vi "REAL worker.vi"(3 "channel":i8) -> (1 "Action running":T1(ring)=enum."pre-reaction")   [LabVIEW 2023]
panel:
  out "Time/min":i32
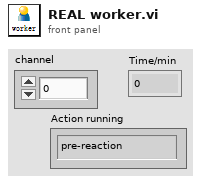
[diagram p1: front panel]
types:
  T1 = enum16{"standby", "pre-reaction", "reaction", "post-reaction", "analysis"}
  T2 = enum16{"check", "scan", "index", "read", "add", "write"}
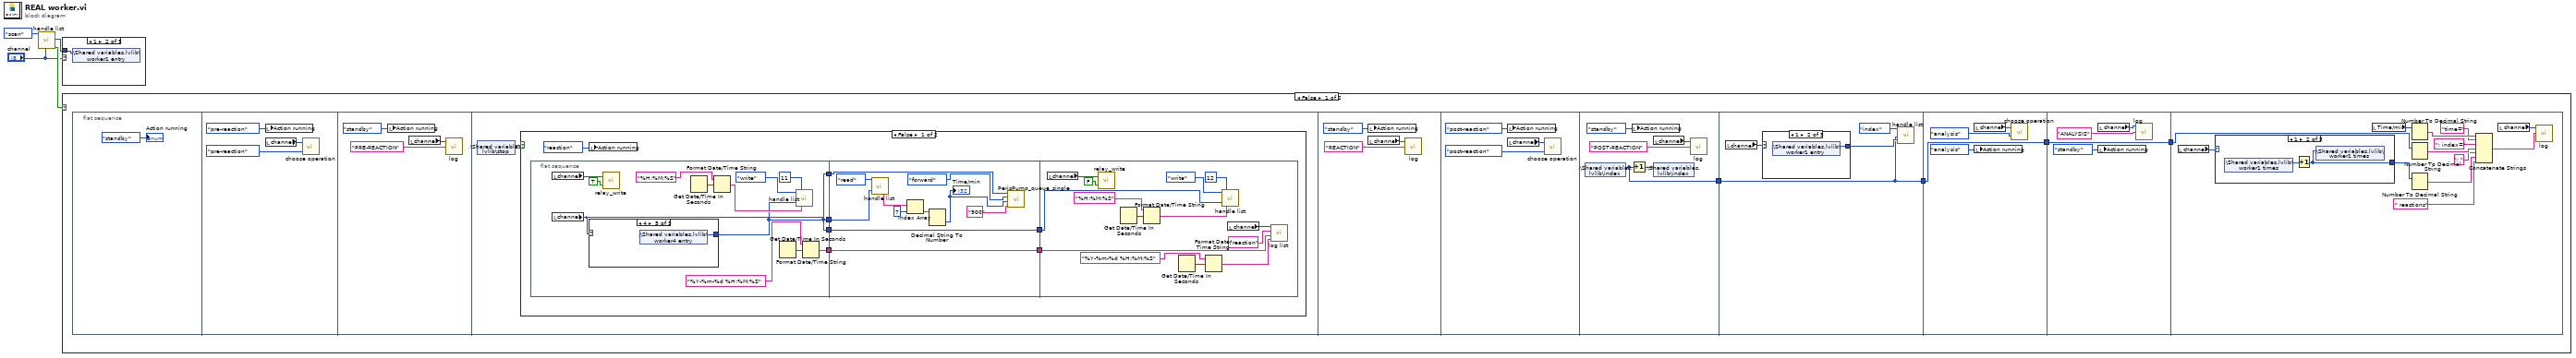
[diagram p0: block diagram]
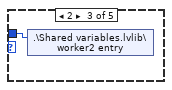
[diagram p3: hidden frame]
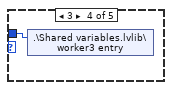
[diagram p4: hidden frame]
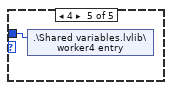
[diagram p5: hidden frame]
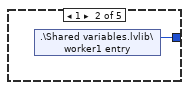
[diagram p7: hidden frame]
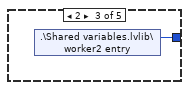
[diagram p8: hidden frame]
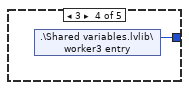
[diagram p9: hidden frame]
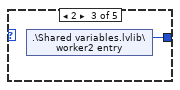
[diagram p12: hidden frame]
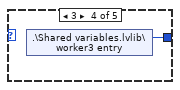
[diagram p13: hidden frame]
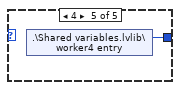
[diagram p14: hidden frame]
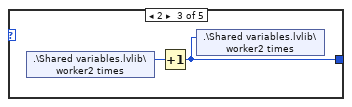
[diagram p16: hidden frame]
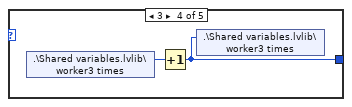
[diagram p17: hidden frame]
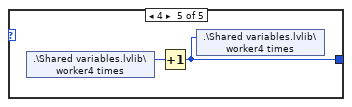
[diagram p18: hidden frame]
diagram:
  n1 = call "handle list.vi"("operation"=T2."scan", "channel"="channel") -> ("output entry"=w1:i32, "done"=w4:bool)  [unwired: 14 in, 2 out]
  n2 = case shown="1" "channel" {
    tunnel: w1 -> [_ w5 w6 w7 w8]
    frame 0, Default {
    }
    frame 1 {
      n3 = shared-variable ".\\Shared variables.lvlib\\worker1 entry"(w5) -> ()  [unwired: 1 in, 1 out]
    }
    frame 2 {
      n4 = shared-variable ".\\Shared variables.lvlib\\worker2 entry"(w6) -> ()  [unwired: 1 in, 1 out]
    }
    frame 3 {
      n5 = shared-variable ".\\Shared variables.lvlib\\worker3 entry"(w7) -> ()  [unwired: 1 in, 1 out]
    }
    frame 4 {
      n6 = shared-variable ".\\Shared variables.lvlib\\worker4 entry"(w8) -> ()  [unwired: 1 in, 1 out]
    }
  }
  n7 = case shown="False" w4 {
    frame False {
      n8 = flat-sequence {
        tunnel: [w75] -> w12
        tunnel: w12 -> [w81]
        tunnel: [w81] -> w10
        tunnel: [w88] -> w11
        tunnel: w10 -> [w88]
        tunnel: [w92] -> w9
        tunnel: w11 -> [w92]
        tunnel: w9 -> [w96]
        frame #0 {
          "Action running" <- T1."standby" ("Action running")
        }
        frame #1 {
          n9 = local write "Action running"(T1."pre-reaction" ("Action running")) -> ()
          n10 = local read "channel"() -> (w15:i8)
          n11 = call "choose operation.vi"("Enum"=T1."pre-reaction", "channel"=w15) -> ()  [unwired: 1 in]
        }
        frame #2 {
          n12 = local write "Action running"(T1."standby" ("Action running")) -> ()
          n13 = local read "channel"() -> (w17:i8)
          n14 = call "log.vi"("worker"=w17, "input string"="PRE-REACTION") -> ()  [unwired: 6 in, 3 out]
        }
        frame #3 {
          n15 = shared-variable ".\\Shared variables.lvlib\\stop"() -> (w20:bool)  [unwired: 1 in, 1 out]
          n16 = case shown="False" w20 {
            frame False {
              n17 = flat-sequence {
                tunnel: [w33] -> w26
                tunnel: [w34] -> w25
                tunnel: [w33] -> w23
                tunnel: [w28] -> w21
                tunnel: w26 -> [w48]
                tunnel: w25 -> [w47]
                tunnel: [w46] -> w24
                tunnel: w23 -> [w46]
                tunnel: [w45] -> w22
                tunnel: w21 -> [w45]
                tunnel: w24 -> [w63]
                tunnel: w22 -> [w60]
                frame #0 {
                  n18 = local read "channel"() -> (w32:i8)
                  n19 = local read "channel"() -> (w34:i8)
                  n20 = case shown="4" w34 {
                    tunnel: [_ w40 w41 w42 w43] -> w33
                    frame 0, Default {
                    }
                    frame 1 {
                      n21 = shared-variable ".\\Shared variables.lvlib\\worker1 entry"() -> (w40:i32)  [unwired: 1 in, 1 out]
                    }
                    frame 2 {
                      n22 = shared-variable ".\\Shared variables.lvlib\\worker2 entry"() -> (w41:i32)  [unwired: 1 in, 1 out]
                    }
                    frame 3 {
                      n23 = shared-variable ".\\Shared variables.lvlib\\worker3 entry"() -> (w42:i32)  [unwired: 1 in, 1 out]
                    }
                    frame 4 {
                      n24 = shared-variable ".\\Shared variables.lvlib\\worker4 entry"() -> (w43:i32)  [unwired: 1 in, 1 out]
                    }
                  }
                  n25 = call "relay_write.vi"("on/off"=TRUE, "No."=w32) -> ()  [unwired: 1 out]
                  n26 = Get Date/Time In Seconds() -> (seconds since 1Jan1904=w39:timestamp)
                  n27 = Format Date/Time String(time format string (%c)="%H:%M:%S", seconds (now)=w39) -> (date/time string=w37:string)  [unwired: 1 in]
                  n28 = Get Date/Time In Seconds() -> (seconds since 1Jan1904=w30:timestamp)
                  n29 = call "handle list.vi"("operation"=T2."write", "input entry"=w33, "colume"=11, "new element/subarray"=w37) -> ()  [unwired: 12 in, 4 out]
                  n30 = Format Date/Time String(time format string (%c)="%Y-%m-%d %H:%M:%S", seconds (now)=w30) -> (date/time string=w28:string)  [unwired: 1 in]
                }
                frame #1 {
                  n31 = call "handle list.vi"("operation"=T2."read", "input entry"=w48) -> ("subarray"=w53:string[])  [unwired: 14 in, 3 out]
                  n32 = Index Array(array=w53, index=7) -> (element=w50:string)
                  n33 = Decimal String To Number(string=w50) -> (number=w44:i32)  [unwired: 2 in, 1 out]
                  "Time/min" <- w44
                  n34 = call "PerisPump_queue_single.vi"("Step"="900", "Time/min"=w44, "First step"=enum16{"forward", "backward"}."forward", "Address"=w47) -> ()  [unwired: 7 in, 1 out]
                }
                frame #2 {
                  n35 = local read "channel"() -> (w61:i8)
                  n36 = call "relay_write.vi"("on/off"=FALSE, "No."=w61) -> ()  [unwired: 1 out]
                  n37 = Get Date/Time In Seconds() -> (seconds since 1Jan1904=w68:timestamp)
                  n38 = Format Date/Time String(time format string (%c)="%H:%M:%S", seconds (now)=w68) -> (date/time string=w66:string)  [unwired: 1 in]
                  n39 = Get Date/Time In Seconds() -> (seconds since 1Jan1904=w57:timestamp)
                  n40 = Format Date/Time String(time format string (%c)="%Y-%m-%d %H:%M:%S", seconds (now)=w57) -> (date/time string=w55:string)  [unwired: 1 in]
                  n41 = call "handle list.vi"("operation"=T2."write", "input entry"=w63, "colume"=12, "new element/subarray"=w66) -> ()  [unwired: 12 in, 4 out]
                  n42 = local read "channel"() -> (w59:i8)
                  n43 = call "log list.vi"("end"=w55, "start"=w60, "operaton"="reaction", "worker"=w59) -> ()  [unwired: 7 in, 1 out]
                }
              }
              n44 = local write "Action running"(T1."reaction" ("Action running")) -> ()
            }
            frame True {
            }
          }
        }
        frame #4 {
          n45 = local write "Action running"(T1."standby" ("Action running")) -> ()
          n46 = local read "channel"() -> (w69:i8)
          n47 = call "log.vi"("worker"=w69, "input string"="REACTION") -> ()  [unwired: 6 in, 3 out]
        }
        frame #5 {
          n48 = local write "Action running"(T1."post-reaction" ("Action running")) -> ()
          n49 = local read "channel"() -> (w73:i8)
          n50 = call "choose operation.vi"("Enum"=T1."post-reaction", "channel"=w73) -> ()  [unwired: 1 in]
        }
        frame #6 {
          n51 = shared-variable ".\\Shared variables.lvlib\\index"() -> (w75:i8)  [unwired: 1 in, 1 out]
          n52 = Increment(x=w75) -> (x+1=w76:i8)
          n53 = local write "Action running"(T1."standby" ("Action running")) -> ()
          n54 = local read "channel"() -> (w77:i8)
          n55 = shared-variable ".\\Shared variables.lvlib\\index"(w76) -> ()  [unwired: 1 in, 1 out]
          n56 = call "log.vi"("worker"=w77, "input string"="POST-REACTION") -> ()  [unwired: 6 in, 3 out]
        }
        frame #7 {
          n57 = local read "channel"() -> (w82:i8)
          n58 = case shown="1" w82 {
            tunnel: [_ w84 w85 w86 w87] -> w83
            frame 0, Default {
            }
            frame 1 {
              n59 = shared-variable ".\\Shared variables.lvlib\\worker1 entry"() -> (w84:i32)  [unwired: 1 in, 1 out]
            }
            frame 2 {
              n60 = shared-variable ".\\Shared variables.lvlib\\worker2 entry"() -> (w85:i32)  [unwired: 1 in, 1 out]
            }
            frame 3 {
              n61 = shared-variable ".\\Shared variables.lvlib\\worker3 entry"() -> (w86:i32)  [unwired: 1 in, 1 out]
            }
            frame 4 {
              n62 = shared-variable ".\\Shared variables.lvlib\\worker4 entry"() -> (w87:i32)  [unwired: 1 in, 1 out]
            }
          }
          n63 = call "handle list.vi"("operation"=T2."index", "index"=w81, "input entry"=w83) -> ()  [unwired: 13 in, 4 out]
        }
        frame #8 {
          n64 = local read "channel"() -> (w90:i8)
          n65 = local write "Action running"(T1."analysis" ("Action running")) -> ()
          n66 = call "choose operation.vi"("Enum"=T1."analysis", "channel"=w90) -> ()  [unwired: 1 in]
        }
        frame #9 {
          n67 = local read "channel"() -> (w93:i8)
          n68 = local write "Action running"(T1."standby" ("Action running")) -> ()
          n69 = call "log.vi"("worker"=w93, "input string"="ANALYSIS") -> ()  [unwired: 6 in, 3 out]
        }
        frame #10 {
          n70 = local read "channel"() -> (w104:i8)
          n71 = case shown="1" w104 {
            tunnel: [_ w109 w111 w113 w115] -> w103
            frame 0, Default {
            }
            frame 1 {
              n72 = shared-variable ".\\Shared variables.lvlib\\worker1 times"() -> (w110:i8)  [unwired: 1 in, 1 out]
              n73 = Increment(x=w110) -> (x+1=w109:i8)
              n74 = shared-variable ".\\Shared variables.lvlib\\worker1 times"(w109) -> ()  [unwired: 1 in, 1 out]
            }
            frame 2 {
              n75 = shared-variable ".\\Shared variables.lvlib\\worker2 times"() -> (w112:i8)  [unwired: 1 in, 1 out]
              n76 = Increment(x=w112) -> (x+1=w111:i8)
              n77 = shared-variable ".\\Shared variables.lvlib\\worker2 times"(w111) -> ()  [unwired: 1 in, 1 out]
            }
            frame 3 {
              n78 = shared-variable ".\\Shared variables.lvlib\\worker3 times"() -> (w114:i8)  [unwired: 1 in, 1 out]
              n79 = Increment(x=w114) -> (x+1=w113:i8)
              n80 = shared-variable ".\\Shared variables.lvlib\\worker3 times"(w113) -> ()  [unwired: 1 in, 1 out]
            }
            frame 4 {
              n81 = shared-variable ".\\Shared variables.lvlib\\worker4 times"() -> (w116:i8)  [unwired: 1 in, 1 out]
              n82 = Increment(x=w116) -> (x+1=w115:i8)
              n83 = shared-variable ".\\Shared variables.lvlib\\worker4 times"(w115) -> ()  [unwired: 1 in, 1 out]
            }
          }
          n84 = local read "Time/min"() -> (w99:i32)
          n85 = Number To Decimal String(number=w99) -> (decimal integer string=w98:string)  [unwired: 1 in]
          n86 = Number To Decimal String(number=w96) -> (decimal integer string=w101:string)  [unwired: 1 in]
          n87 = Number To Decimal String(number=w103) -> (decimal integer string=w108:string)  [unwired: 1 in]
          n88 = Concatenate Strings("time=" ("string"), w98, "; index=" ("string"), w101, "; " ("string"), w108, " reactions" ("string")) -> (w106:string)
          n89 = local read "channel"() -> (w105:i8)
          n90 = call "log.vi"("worker"=w105, "input string"=w106) -> ()  [unwired: 6 in, 3 out]
        }
      }
    }
    frame True {
    }
  }
